vi "XYZ_Pos_to_string.vi"(1 "Position label":string, 2 "Z":dbl format="%.2f", 3 "Y":dbl format="%.2f", 4 "X":dbl format="%.2f") -> (0 "Output string":string)   [LabVIEW 2011]
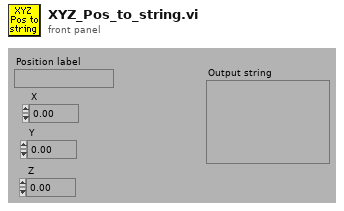
[diagram p1: front panel]
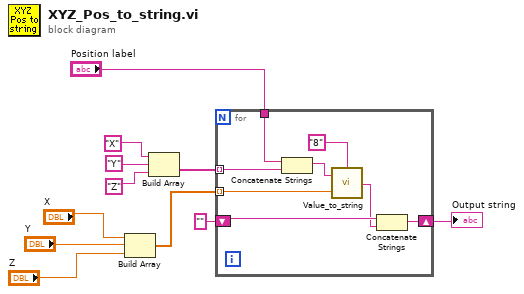
[diagram p0: block diagram]
diagram:
  n1 = Build Array("X", "Y", "Z") -> (w4:dbl[])
  n2 = Build Array("X", "Y", "Z") -> (w10:string[])
  n3 = for {
    tunnel: "Position label" -> [w13]
    tunnel: w10 -> [w19] mode=indexing
    tunnel: w4 -> [w17] mode=indexing
    shift-right: [w14] -> w5
    shift-left: "" -> [w16]
    n4 = Concatenate Strings(w13, w19) -> (w18:string)
    n5 = call "Value_to_string.vi"("precision"="8", "Value"=w17, "Label for value"=w18) -> ("Output string"=w15:string)
    n6 = Concatenate Strings(w16, w15) -> (w14:string)
  }
  "Output string" <- w5
